vi "Motor_Output.vi"(0 "Can_Door":bool, 3 "Ref_Num":T27, 4 "Can_Tip_Flip":bool, 5 "Can_Tip_Arm":bool, 6 "Infeed_Pneu":bool, 7 "Ele_Outfeed":dbl, 8 "Arm_Sol_Pos":bool, 9 "Ele_Lift":dbl, 10 "Intake":dbl, 11 "Arm_Sol_Ext":bool) -> ()   [LabVIEW 2014]
uses:
  <vilib>/Rock Robotics/WPI/Joystick/WPI_JoystickDevRef.ctl
  <vilib>/Rock Robotics/WPI/Joystick/WPI_JoystickDeviceEnum.ctl
  <vilib>/Rock Robotics/WPI/RobotDrive/WPI_RobotDriveDevRef.ctl
  <vilib>/Rock Robotics/WPI/MotorControl/WPI_MotorControlDeviceRef.ctl
  <vilib>/Rock Robotics/WPI/MotorControl/WPI_MotorControlType.ctl
  <vilib>/Rock Robotics/SystemInterfaces/Typedef/FPGA_TypedefDigitalModule.ctl
  <vilib>/Rock Robotics/SystemInterfaces/DIO/FPGA_DIOPWMChannel.ctl
  <vilib>/Rock Robotics/WPI/PWM/WPI_PWMDeadband.ctl
  <vilib>/Rock Robotics/WPI/CAN/Jaguar/SubVIs/WPI_CANJaguar_ControlMode.ctl
  <vilib>/Rock Robotics/WPI/CAN/TalonSRX/WPI_CANTalonSRX_APIControlMode.ctl
  <vilib>/Rock Robotics/WPI/PWM/WPI_PWMTransform_ConPane.ctl
  <vilib>/Rock Robotics/WPI/Encoder/WPI_EncoderDevRef.ctl
  <vilib>/Rock Robotics/SystemInterfaces/Encoder/FPGA_EncoderIdx.ctl
  <vilib>/Rock Robotics/SystemInterfaces/Counter/FPGA_CounterCtrSystemIndex.ctl
  <vilib>/Rock Robotics/WPI/Encoder/WPI_EncoderType.ctl
  <vilib>/Rock Robotics/WPI/Switch/WPI_SwitchDevRef.ctl
  <vilib>/Rock Robotics/SystemInterfaces/DIO/FPGA_DIOChannel.ctl
  <vilib>/Rock Robotics/WPI/AnalogChannel/WPI_AnalogChannelDevRef.ctl
  <vilib>/Rock Robotics/SystemInterfaces/Typedef/FPGA_TypedefAnalogModule.ctl
  <vilib>/Rock Robotics/SystemInterfaces/AI/FPGA_AIChannel.ctl
  AdaIMU roboRIO/IMUDevRef.ctl
  <vilib>/Rock Robotics/SystemInterfaces/i2clib/i2c_bus.ctl
  <vilib>/Rock Robotics/WPI/Compressor/WPI_CompressorDevRef.ctl
  <vilib>/Rock Robotics/WPI/Solenoid/WPI_SolenoidDevRef.ctl
  <vilib>/Rock Robotics/WPI/Solenoid/WPI_SolenoidChannel.ctl
  <vilib>/Rock Robotics/WPI/Solenoid/WPI_SolenoidValue.ctl
  <vilib>/Rock Robotics/WPI/Solenoid/WPI_SolenoidSetEnum.vi
panel:
  # "Motor Controls"
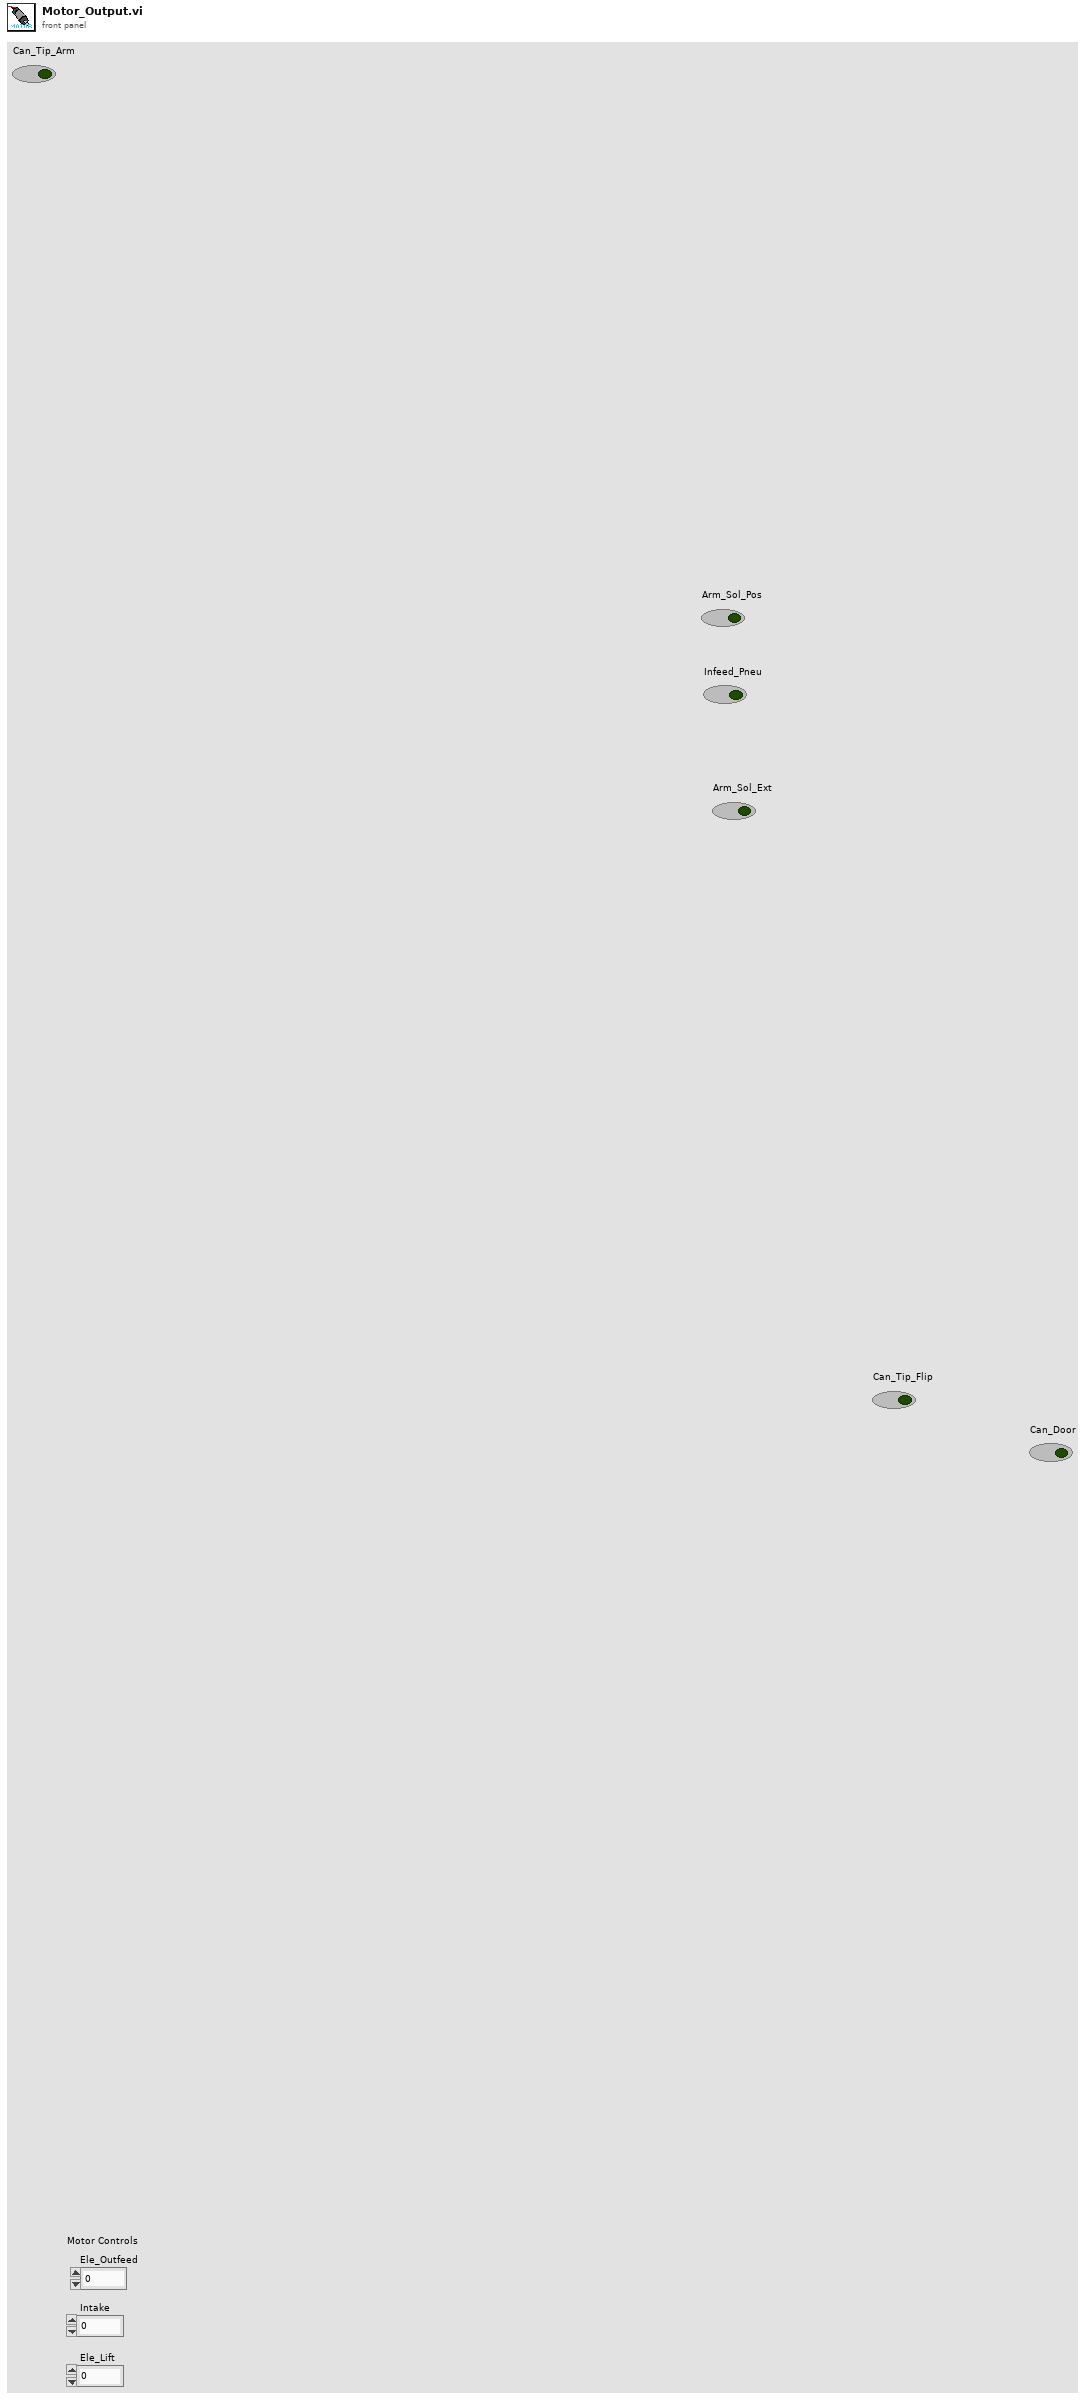
[diagram p1: front panel]
types:
  T1 = typedef "WPI_JoystickDevRef.ctl" = cluster{"Device":T2}
  T2 = typedef "WPI_JoystickDeviceEnum.ctl" = enum16{"USB 0", "USB 1", "USB 2", "USB 3", "USB 4", "USB 5"}
  T3 = typedef "WPI_RobotDriveDevRef.ctl" = cluster{"DevStatus":errorcluster, "Motors[]":T4[], "Square Inputs":bool, "Max Output":dbl}
  T4 = typedef "WPI_MotorControlDeviceRef.ctl" = cluster{"DeviceStatus":errorcluster, "Type":T5, "PWM":cluster{"Controller":T6, "PWM Channel":T7, "DeadBand":T8}, "CAN":cluster{"Device Number":u8, "Control Mode":T9, "Semaphore":T10, "Max Vout":dbl, "TalonSRX Control Mode":T11}, "Invert":bool, "TransformRef":T12, "InvTransformRef":T12}
  T5 = typedef "WPI_MotorControlType.ctl" = enum16{"PWM", "CAN", "CANTalonSRX"}
  T6 = typedef "FPGA_TypedefDigitalModule.ctl" = enum16{"Controller 1"}
  T7 = typedef "FPGA_DIOPWMChannel.ctl" = enum8{"PWM 0", "PWM 1", "PWM 2", "PWM 3", "PWM 4", "PWM 5", "PWM 6", "PWM 7", "PWM 8", "PWM 9", "PWM MXP 0", "PWM MXP 1", "PWM MXP 2", "PWM MXP 3", "PWM MXP 4", "PWM MXP 5", "PWM MXP 6", "PWM MXP 7", "PWM MXP 8", "PWM MXP 9", "Invalid"}
  T8 = typedef "WPI_PWMDeadband.ctl" = cluster{"Name":string, "maxPositivePwm":i32, "minPositivePwm":i32, "centerPwm":i32, "maxNegativePwm":i32, "minNegativePwm":i32, "angularRange":u16}
  T9 = typedef "WPI_CANJaguar_ControlMode.ctl" = enum8{"Percent VBus", "Current", "Speed", "Position", "Voltage"}
  T10 = typedef "Semaphore RefNum" = refnum<k1>
  T11 = typedef "WPI_CANTalonSRX_APIControlMode.ctl" = enum8{"Percent VBus", "Speed", "Position", "Slave", "Unchanged / Invalid"}
  T12 = typedef "WPI_PWMTransform_ConPane.ctl" = refnum<vi>
  T13 = typedef "WPI_EncoderDevRef.ctl" = cluster{"DevStatus":errorcluster, "EncoderIndex":T14, "CounterIndex":T15, "DistancePerCount":dbl, "Decoding Type":T16}
  T14 = typedef "FPGA_EncoderIdx.ctl" = enum8{"Enc 0", "Enc 1", "Enc 2", "Enc 3", "Enc 4", "Enc 5", "Enc 6", "Enc 7", "Invalid"}
  T15 = typedef "FPGA_CounterCtrSystemIndex.ctl" = enum8{"Ctr 0", "Ctr 1", "Ctr 2", "Ctr 3", "Ctr 4", "Ctr 5", "Ctr 6", "Ctr 7", "Invalid"}
  T16 = typedef "WPI_EncoderType.ctl" = enum16{"1x", "2x", "4x"}
  T17 = typedef "WPI_SwitchDevRef.ctl" = cluster{"DevStatus":errorcluster, "DIO Channel":T18, "Controller":T6, "CntIndex":T15, "Normally Closed":bool}
  T18 = typedef "FPGA_DIOChannel.ctl" = enum8{"DIO 0", "DIO 1", "DIO 2", "DIO 3", "DIO 4", "DIO 5", "DIO 6", "DIO 7", "DIO 8", "DIO 9", "DIO MXP 0", "DIO MXP 1", "DIO MXP 2", "DIO MXP 3", "DIO MXP 4", "DIO MXP 5", "DIO MXP 6", "DIO MXP 7", "DIO MXP 8", "DIO MXP 9", "DIO MXP 10", "DIO MXP 11", "DIO MXP 12", "DIO MXP 13", "DIO MXP 14", "DIO MXP 15", "Invalid"}
  T19 = typedef "WPI_AnalogChannelDevRef.ctl" = cluster{"DevStatus":errorcluster, "Controller":T20, "Analog Channel":T21}
  T20 = typedef "FPGA_TypedefAnalogModule.ctl" = enum16{"Controller 1"}
  T21 = typedef "FPGA_AIChannel.ctl" = enum8{"AI 0", "AI 1", "AI 2", "AI 3", "AI MXP 0", "AI MXP 1", "AI MXP 2", "AI MXP 3", "Invalid"}
  T22 = typedef "IMUDevRef.ctl" = cluster{"DevStatus":errorcluster, "Gyro Address":u8, "Gyro Range":u8, "Mean Rates":cluster{"Xmo":dbl, "Ymo":dbl, "Zmo":dbl}, "StdDev Rates":cluster{"Xsdo":dbl, "Ysdo":dbl, "Zsdo":dbl}, "Fast":bool, "Reset":bool, "Accel Address":u8, "Accel Range":u8, "Accel Scale":cluster{"Xscale":dbl, "Yscale":dbl, "Zscale":dbl}, "Mag Address":u8, "Mag Range":u8, "G Sense":bool, "A Sense":bool, "M Sense":bool, "Accel Offset":cluster{"Xzero":dbl, "Yzero":dbl, "Zzero":dbl}, "Motion Thresh":dbl, "Mag Scale":cluster{"Xscale":dbl, "Yscale":dbl, "Zscale":dbl}, "Mag Offset":cluster{"Xzero":dbl, "Yzero":dbl, "Zzero":dbl}, "I2C Bus":T23, "Handle":i32, "Controller":T6, "Anomaly Thresh":dbl, "Local Mag":dbl}
  T23 = typedef "i2c_bus.ctl" = enum16{"I2C On-Board", "I2C MXP", "Invalid"}
  T24 = typedef "WPI_CompressorDevRef.ctl" = cluster{"DevStatus":errorcluster, "Pneumatics Control Module":u8}
  T25 = typedef "WPI_SolenoidDevRef.ctl" = cluster{"DevStatus":errorcluster, "Pneumatics Control Module":u8, "Forward Solenoid Channel":T26, "Reverse Solenoid Channel":T26}
  T26 = typedef "WPI_SolenoidChannel.ctl" = enum8{"Solenoid 0", "Solenoid 1", "Solenoid 2", "Solenoid 3", "Solenoid 4", "Solenoid 5", "Solenoid 6", "Solenoid 7", "Invalid"}
  T27 = cluster{"Joystick":cluster{"Drive_Joystick":T1, "Imp_Joystick":T1}, "Motor":cluster{"Left and Right Motors":T3, "Left_Intake":T4, "Right_Intake":T4, "Elevator_Lift":T4, "Elevator_Arm_Left":T4, "Elevator_Arm_Right":T4}, "Encoder":cluster{"Left_Drive_Speed":T13, "Auto_2_Tote":T17, "Auto_Cans":T17, "Auto_Cans_Delay":T17}, "Analog":cluster{"Tote_Detect_1":T19, "Tote_Detect_2":T19, "Ele_Pos_Yoyo":T19, "Auto_Switch":T19}, "IMU_Reft_Num":T22, "Pneumatics":cluster{"Compressor":T24, "Arm_Sol":T25, "Infeed_Pneu":T25, "Can_Tip_Flip":T25, "Can_Tip_Arm":T25, "Can_Door_Arm":T25, "Arm_Sol_Ext":T25}}
  T28 = typedef "WPI_SolenoidValue.ctl" = enum16{"Off", "On", "Forward", "Reverse"}
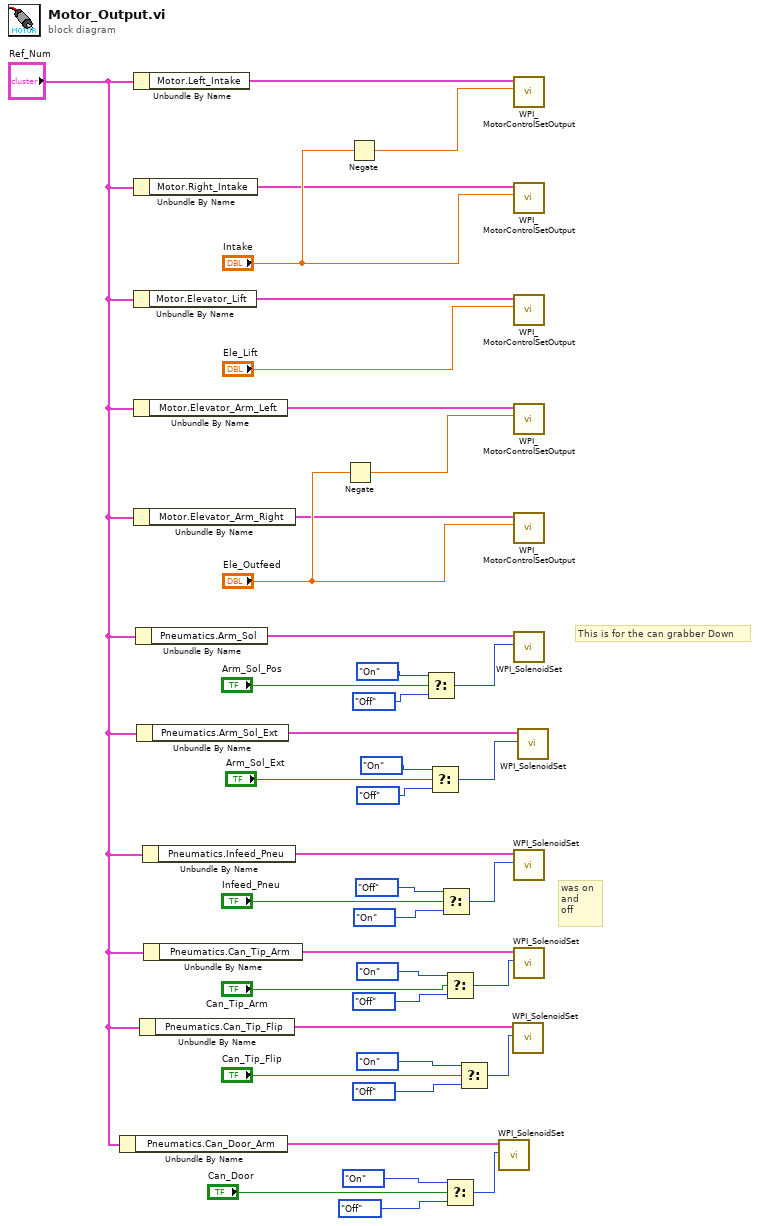
[diagram p0: block diagram]
diagram:
  # "This is for the can grabber Down"
  # "was on \nand \noff"
  n1 = Unbundle By Name("Ref_Num") -> ("Pneumatics.Can_Door_Arm"=w7:T25)
  n2 = Unbundle By Name("Ref_Num") -> ("Motor.Left_Intake"=w36:T4)
  n3 = Unbundle By Name("Ref_Num") -> ("Motor.Right_Intake"=w35:T4)
  n4 = Unbundle By Name("Ref_Num") -> ("Motor.Elevator_Lift"=w34:T4)
  n5 = Unbundle By Name("Ref_Num") -> ("Motor.Elevator_Arm_Left"=w33:T4)
  n6 = Unbundle By Name("Ref_Num") -> ("Motor.Elevator_Arm_Right"=w32:T4)
  n7 = Unbundle By Name("Ref_Num") -> ("Pneumatics.Arm_Sol"=w30:T25)
  n8 = Unbundle By Name("Ref_Num") -> ("Pneumatics.Arm_Sol_Ext"=w3:T25)
  n9 = Unbundle By Name("Ref_Num") -> ("Pneumatics.Can_Tip_Flip"=w20:T25)
  n10 = Unbundle By Name("Ref_Num") -> ("Pneumatics.Infeed_Pneu"=w31:T25)
  n11 = Unbundle By Name("Ref_Num") -> ("Pneumatics.Can_Tip_Arm"=w29:T25)
  n12 = Negate(x="Ele_Outfeed") -> (-x=w40:dbl)
  n13 = Negate(x="Intake") -> (-x=w38:dbl)
  n14 = Select(t=WPI_SolenoidValue."On" ("Value"), s="Arm_Sol_Pos", f=WPI_SolenoidValue."Off" ("Value")) -> (s? t:f=w25:T28)
  n15 = Select(t=WPI_SolenoidValue."On" ("Value"), s="Arm_Sol_Ext", f=WPI_SolenoidValue."Off" ("Value")) -> (s? t:f=w2:T28)
  n16 = Select(t=WPI_SolenoidValue."Off" ("Value"), s="Infeed_Pneu", f=WPI_SolenoidValue."On" ("Value")) -> (s? t:f=w21:T28)
  n17 = Select(t=WPI_SolenoidValue."On" ("Value"), s="Can_Tip_Arm", f=WPI_SolenoidValue."Off" ("Value")) -> (s? t:f=w13:T28)
  n18 = Select(t=WPI_SolenoidValue."On" ("Value"), s="Can_Door", f=WPI_SolenoidValue."Off" ("Value")) -> (s? t:f=w11:T28)
  n19 = Select(t=WPI_SolenoidValue."On" ("Value"), s="Can_Tip_Flip", f=WPI_SolenoidValue."Off" ("Value")) -> (s? t:f=w16:T28)
  n20 = call-poly <vilib>:"WPI_SolenoidSet.vi"("Value"=w11, "SolenoidDevRef"=w7) -> ()  [unwired: 8 in, 2 out]
  n21 = call-poly <vilib>:"WPI_SolenoidSet.vi"("Value"=w16, "SolenoidDevRef"=w20) -> ()  [unwired: 8 in, 2 out]
  n22 = call <vilib>:"WPI_MotorControlSetOutput.vi"("Output"=w38, "MotorControlDevRef"=w36) -> ()  [unwired: 7 in, 3 out]
  n23 = call <vilib>:"WPI_MotorControlSetOutput.vi"("Output"="Intake", "MotorControlDevRef"=w35) -> ()  [unwired: 7 in, 3 out]
  n24 = call <vilib>:"WPI_MotorControlSetOutput.vi"("Output"="Ele_Lift", "MotorControlDevRef"=w34) -> ()  [unwired: 7 in, 3 out]
  n25 = call <vilib>:"WPI_MotorControlSetOutput.vi"("Output"=w40, "MotorControlDevRef"=w33) -> ()  [unwired: 7 in, 3 out]
  n26 = call <vilib>:"WPI_MotorControlSetOutput.vi"("Output"="Ele_Outfeed", "MotorControlDevRef"=w32) -> ()  [unwired: 7 in, 3 out]
  n27 = call-poly <vilib>:"WPI_SolenoidSet.vi"("Value"=w25, "SolenoidDevRef"=w30) -> ()  [unwired: 8 in, 2 out]
  n28 = call-poly <vilib>:"WPI_SolenoidSet.vi"("Value"=w21, "SolenoidDevRef"=w31) -> ()  [unwired: 8 in, 2 out]
  n29 = call-poly <vilib>:"WPI_SolenoidSet.vi"("Value"=w13, "SolenoidDevRef"=w29) -> ()  [unwired: 8 in, 2 out]
  n30 = call-poly <vilib>:"WPI_SolenoidSet.vi"("Value"=w2, "SolenoidDevRef"=w3) -> ()  [unwired: 8 in, 2 out]
